vi "ReadMasterData.vi"(8 "error in (no error)":errorcluster, 11 "Array in":refnum<vi>) -> (0 "error out":errorcluster, 3 "Data":u8[][](array[numeric]))   [LabVIEW 2016]
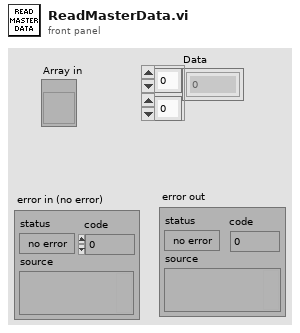
[diagram p1: front panel]
types:
  T1 = typedef "Semaphore RefNum" = refnum<k1>
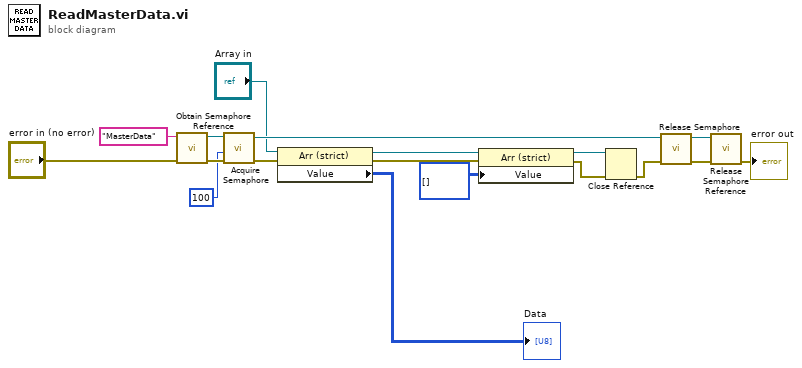
[diagram p0: block diagram]
diagram:
  n1 = call <vilib>:"Obtain Semaphore Reference.vi"("error in (no error)"="error in (no error)", "name (unnamed)"="MasterData") -> ("error out"=w7:errorcluster, "semaphore"=w8:T1)  [unwired: 3 in, 1 out]
  n2 = call <vilib>:"Acquire Semaphore.vi"("error in (no error)"=w7, "ms timeout (-1)"=100, "semaphore"=w8) -> ("error out"=w9:errorcluster, "semaphore out"=w13:T1)  [unwired: 2 in, 1 out]
  n3 = property on="Property Node" class="Arr (strict)"(reference="Array in", error in=w9) -> (reference out=w11:refnum<vi>, error out=w12:errorcluster, "Value"=→"Data":u8[][])
  n4 = property on="Property Node" class="Arr (strict)"(reference=w11, error in=w12, "Value"=u8[][] [] ("Value (Signaling)")) -> (reference out=w15:refnum<vi>, error out=w14:errorcluster)
  n5 = Close Reference(reference=w15, error in (no error)=w14) -> (error out=w16:errorcluster)
  n6 = call <vilib>:"Release Semaphore.vi"("error in (no error)"=w16, "semaphore"=w13) -> ("error out"=w17:errorcluster, "semaphore out"=w18:T1)  [unwired: 4 in]
  n7 = call <vilib>:"Release Semaphore Reference.vi"("error in (no error)"=w17, "semaphore"=w18) -> ("error out"=→"error out":errorcluster)  [unwired: 8 in, 1 out]
